vi "FormatDouble.vi"(1 "double":dbl) -> (0 "value":string)   [LabVIEW 2014, in "Raspberry Pi Compatible Compiler for LabVIEW.lvlib" / "PythonConfiguration.lvclass"]
uses:
  PythonConfiguration.lvclass
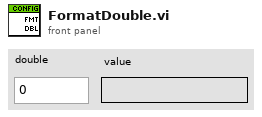
[diagram p1: front panel]
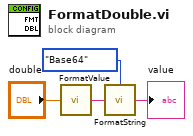
[diagram p0: block diagram]
diagram:
  n1 = call "FormatValue.vi"("value"="double") -> ("value"=w3:string)
  n2 = call "FormatString.vi"("String"=w3, "string encoding"=enum16{"None", "Base64"}."Base64") -> ("value"=→"value":string)
